vi "SetAttributeViInt32_SA-Gating_Sweep.vi"(7 "AttributeValue":i32 format="%.0g", 8 "error in (no error)":errorcluster {"code" format="%.0x"}, 9 "AttributeID":u32(ring)=1150537 items=["SA_GATING_DELAY_COMPENSATION"=1150537, "SA_GATING_METHOD"=1150529, "SA_GATING_SOURCE"=1150531, "SA_GATING_TYPE"=1150532, "SA_LISTSWEEP_FREQUENCY_SYNTHESIS"=1150639, "SA_LISTSWEEP_TRIGGER_SLOPE"=1150657, "SA_LISTSWEEP_TRIGGER_SOURCE"=1150658, "SA_SWEEPCOUPLING_BANDWIDTH_SHAPE"=1150730, "SA_SWEEPCOUPLING_BANDWIDTH_TYPE"=1150731, "SA_SWEEPCOUPLING_SWEEP_POINTS"=1150724, "SA_SWEEPCOUPLING_SWEEP_TIME_AUTO_RULES"=1150732, "SA_SWEEPCOUPLING_SWEEP_TYPE_AUTO_RULES"=1150728, "SA_SWEEPCOUPLING_SWEEP_TYPE"=1150734], 11 "instrument handle":refnum<k15>) -> (0 "error out":errorcluster {"code" format="%.0x"}, 3 "instrument handle out":refnum<k15>)   [LabVIEW 2009, in "Keysight XSAn.lvlib"]
doc: "Sets an Int32 attribute from the instrument driver.\nThe following Attributes are supported:\n\nSA_GATING_DELAY_COMPENSATION\nSA_GATING_METHOD\nSA_GATING_SOURCE\nSA_GATING_TYPE\nSA_LISTSWEEP_FREQUENCY_SYNTHESIS\nSA_LISTSWEEP_TRIGGER_SLOPE\nSA_LISTSWEEP_TRIGGER_SOURCE\nSA_SWEEPCOUPLING_BANDWIDTH_SHAPE\nSA_SWEEPCOUPLING_BANDWIDTH_TYPE\nSA_SWEEPCOUPLING_SWEEP_POINTS\nSA_SWEEPCOUPLING_SWEEP_TIME_AUTO_RULES\nSA_SWEEPCOUPLING_SWEEP_TYPE_AUTO_RULES\nSA_SWEEPCOUPLING_SWEEP_TYPE"
uses:
  <instrlib>/Keysight XSAn/Keysight XSAn.lvlib
  AgXSAn.dll
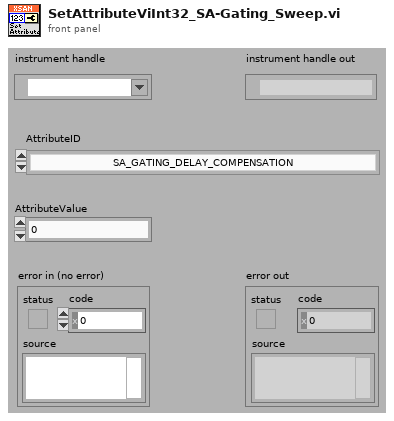
[diagram p1: front panel]
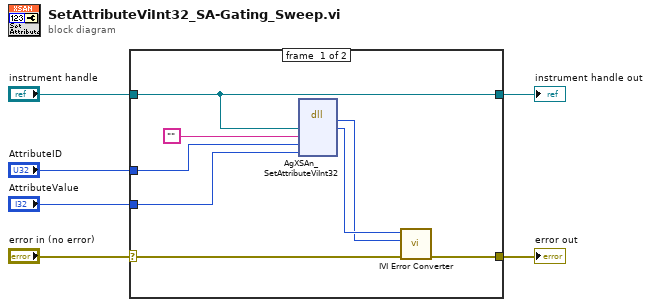
[diagram p0: block diagram]
diagram:
  n1 = case shown="No Error" "error in (no error)" {
    selector: "error in (no error)" -> [w12 w16]
    tunnel: [w11 w16] -> w6
    tunnel: "instrument handle" -> [w8 w15]
    tunnel: "AttributeID" -> [w10 _]
    tunnel: "AttributeValue" -> [w9 _]
    tunnel: [w8 w15] -> w1
    frame #0 {
      n2 = dll-call lib="AgXSAn**.dll" fn="AgXSAn_SetAttributeViInt32"("Vi"=w8, "RepCapIdentifier"="", "AttributeID"=w10, "AttributeValue"=w9) -> ("return type"=w13:i32, "Vi"=w14:u32)  [unwired: 6 in, 2 out]
      n3 = call <instrlib>:"IVI Error Converter.vi"("error in (no error)"=w12, "IVI error code (0)"=w13, "instrument handle"=w14) -> ("error out"=w11:errorcluster)  [unwired: 7 in, 1 out]
    }
    frame #1 {
    }
  }
  "error out" <- w6
  "instrument handle out" <- w1
